vi "StartPanelUpdates.vi"(7 "Ignore Error In":bool, 8 "Error In":errorcluster, 11 "VI Refnum":refnum<vi>) -> (0 "Error Out":errorcluster)   [LabVIEW 2017, in "Client.lvlib" / "UI_API.lvlib"]
uses:
  UI_API.lvlib
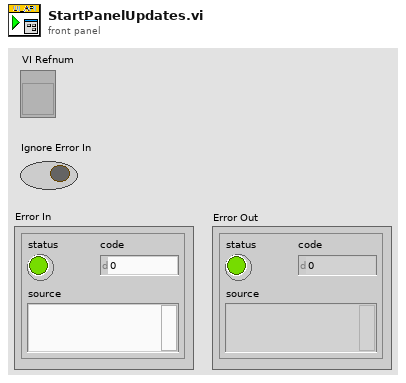
[diagram p1: front panel]
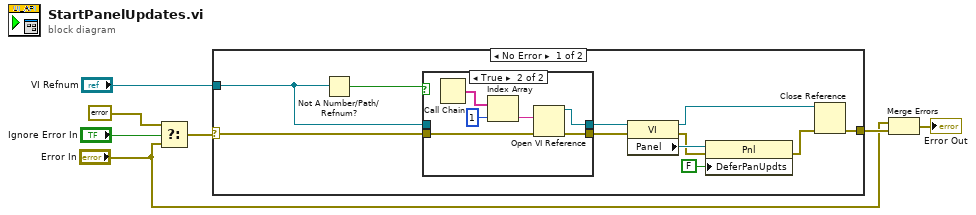
[diagram p0: block diagram]
diagram:
  n1 = Select(t=errorcluster {"status"=FALSE, "code"=0, "source"=""} ("error constant"), s="Ignore Error In", f="Error In") -> (s? t:f=w6:errorcluster)
  n2 = case shown="No Error" w6 {
    selector: w6 -> [w18 w27]
    tunnel: [w10 w27] -> w3
    tunnel: "VI Refnum" -> [w8 _]
    frame No Error {
      n3 = Not A Number/Path/Refnum?(number/path/refnum=w8) -> (NaN/Path/Refnum?=w9:bool)
      n4 = case shown="True" w9 {
        tunnel: w18 -> [w19 w23]
        tunnel: [w19 w22] -> w17
        tunnel: [w20 w21] -> w16
        tunnel: w8 -> [w20 _]
        frame False {
        }
        frame True {
          n5 = Call Chain() -> (call chain=w26:string[])
          n6 = Index Array(array=w26, index=1) -> (element=w24:string)
          n7 = Open VI Reference(vi path=w24, error in (no error)=w23) -> (vi reference=w21:refnum<vi>, error out=w22:errorcluster)  [unwired: 4 in]
        }
      }
      n8 = property class="VI"(reference=w16, error in=w17) -> (reference out=w12:refnum<vi>, error out=w14:errorcluster, "Panel"=w15:refnum<vi>)
      n9 = property class="Pnl"(reference=w15, error in=w14, "DeferPanUpdts"=FALSE ("Defer Panel Updates")) -> (error out=w11:errorcluster)  [unwired: 1 out]
      n10 = Close Reference(reference=w12, error in (no error)=w11) -> (error out=w10:errorcluster)
    }
    frame Error {
    }
  }
  n11 = Merge Errors("Error In", w3) -> (→"Error Out":errorcluster)
